vi "PM100D_Zeroing.vi"(5 "VISA In":refnum<visa-resource-name>) -> (1 "ZeroValue":dbl)   [LabVIEW 2011]
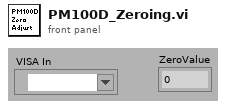
[diagram p1: front panel]
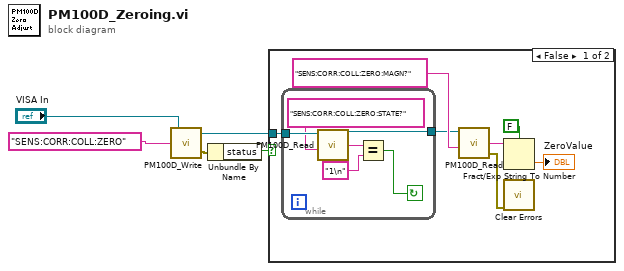
[diagram p0: block diagram]
diagram:
  n1 = call "PM100D_Write.vi"("Command"="SENS:CORR:COLL:ZERO", "VISA in"="VISA In") -> ("error out"=w2:errorcluster, "VISA out"=w5:refnum<visa-resource-name>)  [unwired: 1 in]
  n2 = Unbundle By Name(w2) -> ("status"=w1:bool)
  n3 = case shown="False" w1 {
    tunnel: w5 -> [w10 _]
    frame False {
      n4 = while {
        tunnel: w10 -> [w18]
        tunnel: [w13] -> w11
        stop <- w14 continue-if-true
        n5 = call "PM100D_Read.vi"("Command"="SENS:CORR:COLL:ZERO:STATE?", "VISA in"=w18) -> ("ReadValue"=w16:string, "VISA out"=w13:refnum<visa-resource-name>)  [unwired: 2 in, 1 out]
        n6 = Equal?(x=w16, y="1\n") -> (x = y?=w14:bool)
      }
      n7 = call "PM100D_Read.vi"("Command"="SENS:CORR:COLL:ZERO:MAGN?", "VISA in"=w11) -> ("error out"=w6:errorcluster, "ReadValue"=w9:string)  [unwired: 2 in, 1 out]
      n8 = Fract/Exp String To Number(use system decimal point (T)=FALSE, string=w9) -> (number=→"ZeroValue":dbl)  [unwired: 2 in, 1 out]
      n9 = call <vilib>:"Clear Errors.vi"("error in (no error)"=w6) -> ()  [unwired: 6 in, 1 out]
    }
    frame True {
    }
  }
